vi "tutorial_07.vi"() -> ()   [LabVIEW 2021]
panel:
  out "Média 5 últimas medidas":dbl
  in  "Input":dbl(knob) scale=0.0..100.0
  in  "Temp Scale":bool
  out "Temp History":dbl(graph)
  in  "Power":bool
  # "ON"
  # "OFF"
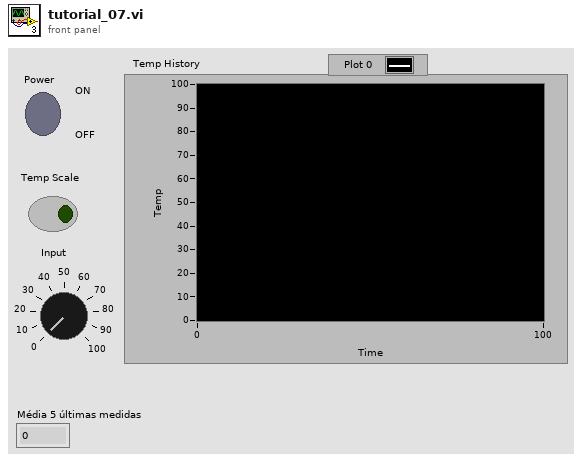
[diagram p1: front panel]
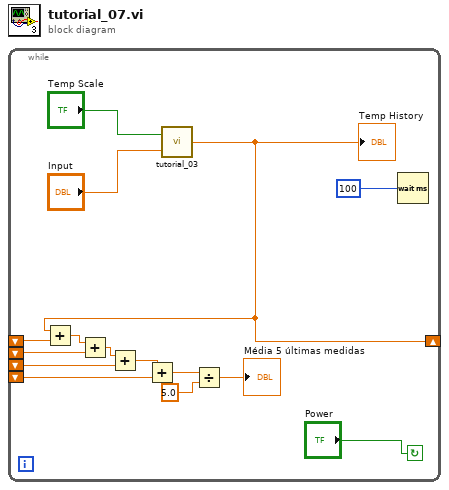
[diagram p0: block diagram]
diagram:
  n1 = while {
    shift-right: [w1] -> _
    shift-left: _ -> [w5]
    shift-left: _ -> [w11]
    shift-left: _ -> [w7]
    shift-left: _ -> [w8]
    stop <- "Power" continue-if-true
    n2 = call "tutorial_03.vi"("Knob"="Input", "Temp Scale"="Temp Scale") -> ("Thermometer"=w1:dbl)
    "Temp History" <- w1
    n3 = Add(x=w1, y=w11) -> (x+y=w9:dbl)
    n4 = Add(x=w9, y=w8) -> (x+y=w10:dbl)
    n5 = Add(x=w10, y=w7) -> (x+y=w6:dbl)
    n6 = Add(x=w6, y=w5) -> (x+y=w4:dbl)
    n7 = Divide(x=w4, y=5.0 ("x/y")) -> (x/y=→"Média 5 últimas medidas":dbl)
    n8 = Wait (ms)(milliseconds to wait=u32 100 ("millisecond timer value")) -> ()  [unwired: 1 out]
  }
